vi "Helper Files_dialog messages.vi"(11 "Why are we here?":T1) -> (2 "Main Msg":string, 3 "Title Message":string)   [LabVIEW 2023]
doc: "Build tiotle and message text for BundleMagic setup dialog based the reason the dialog has been called."
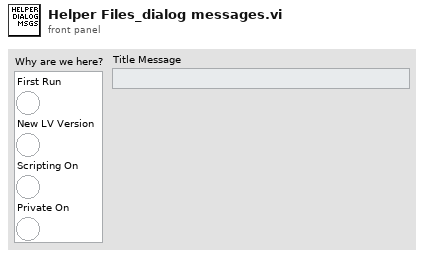
[diagram p1: front panel]
types:
  T1 = cluster{"First Run":bool, "New LV Version":bool, "Scripting On":bool, "Private On":bool}
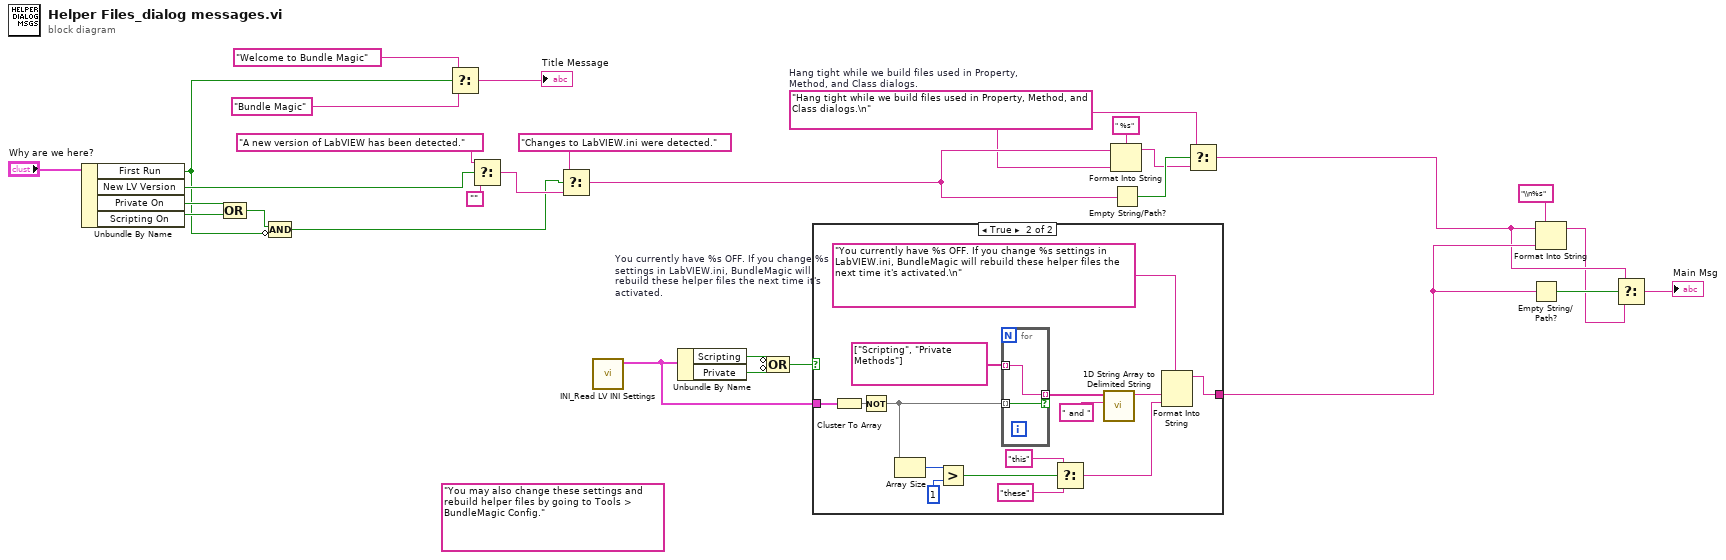
[diagram p0: block diagram]
diagram:
  (unwired) "You may also change these settings and rebuild helper files by going to Tools > BundleMagic Config."
  w9 = "Hang tight while we build files used in Property, Method, and Class dialogs.\n"  # Hang tight while we build files used in Property, Method, and Class dialogs.
  n1 = Unbundle By Name("Why are we here?") -> ("First Run"=w2:bool, "New LV Version"=w25:bool, "Private On"=w5:bool, "Scripting On"=w4:bool)
  n2 = Compound Arithmetic op=OR(w5, w4) -> (w1:bool)
  n3 = Compound Arithmetic op=AND(w1, invert w2) -> (w3:bool)
  n4 = Select(t="Welcome to Bundle Magic", s=w2, f="Bundle Magic") -> (s? t:f=→"Title Message":string)
  n5 = Select(t="A new version of LabVIEW has been detected.", s=w25, f="") -> (s? t:f=w21:string)
  n6 = Select(t="Changes to LabVIEW.ini were detected.", s=w3, f=w21) -> (s? t:f=w10:string)
  n7 = call "INI_Read LV INI Settings.vi"() -> ("LabVIEW INI Settings"=w29:cluster{"Scripting":bool, "Private":bool})  [unwired: 10 in, 1 out]
  n8 = Unbundle By Name(w29) -> ("Scripting"=w8:bool, "Private"=w7:bool)
  n9 = Compound Arithmetic op=OR(invert w8, invert w7) -> (w6:bool)
  n10 = case shown="True" w6 {
    tunnel: w29 -> [_ w39]
    tunnel: [_ w32] -> w15
    frame False {
    }
    frame True {
      w40 = "You currently have %s OFF. If you change %s settings in LabVIEW.ini, BundleMagic will rebuild these helper files the next time it's activated.\n"  # You currently have %s OFF. If you change %s settings in LabVIEW.ini, BundleMagic will rebuild these helper files the next time it's activated.
      n11 = Cluster To Array(cluster=w39) -> (array=w37:bool[])
      n12 = Not(x=w37) -> (.not. x?=w30:bool[])
      n13 = Array Size(array=w30) -> (size(s)=w38:i32)
      n14 = Greater?(x=w38, y=1) -> (0:w31:bool)
      n15 = for {
        tunnel: string[] ["Scripting", "Private Methods"] -> [w46] mode=indexing
        tunnel: w30 -> [w45] mode=indexing
        tunnel: [w46] -> w43 mode=indexing if=w45
      }
      n16 = Select(t="this" ("delimiter"), s=w31, f="these" ("delimiter")) -> (s? t:f=w33:string)
      n17 = call <vilib>:"1D String Array to Delimited String.vi"("delimiter"=" and ", "string array"=w43) -> ("delimited string"=w41:string)  [unwired: 9 in]
      n18 = Format Into String(format string=w40, w41, w33) -> (resulting string=w32:string)  [unwired: 2 in, 1 out]
    }
  }
  n19 = Format Into String(format string=" %s", initial string=w10, w9) -> (resulting string=w17:string)  [unwired: 1 in, 1 out]
  n20 = Empty String/Path?(string/path=w10) -> (empty?=w18:bool)
  n21 = Select(t=w9, s=w18, f=w17) -> (s? t:f=w13:string)
  n22 = Empty String/Path?(string/path=w15) -> (empty?=w14:bool)
  n23 = Format Into String(format string="\\n%s", initial string=w13, w15) -> (resulting string=w12:string)  [unwired: 1 in, 1 out]
  n24 = Select(t=w13, s=w14, f=w12) -> (s? t:f=→"Main Msg":string)
